vi "checkvisionok.vi"(10 "ResultOut":string[][](array[string])) -> (2 "VisionOK":bool)   [LabVIEW 2019]
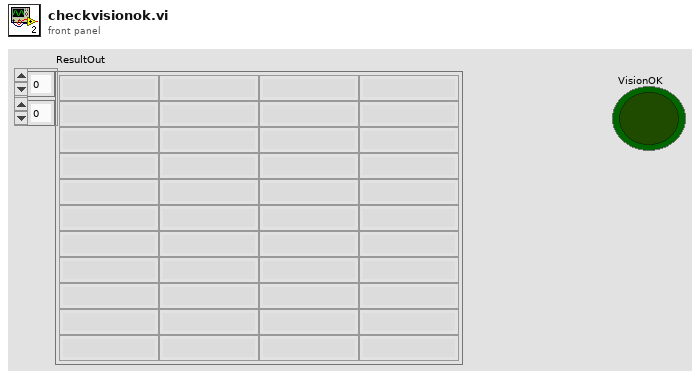
[diagram p1: front panel]
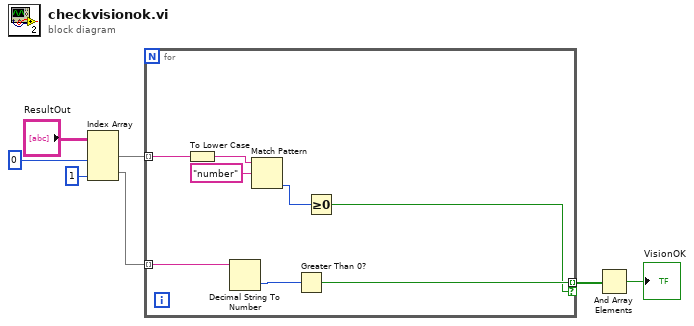
[diagram p0: block diagram]
diagram:
  n1 = Index Array(array="ResultOut", index (col) #1=0 ("disabled index (col)"), index (col) #2=1 ("index (col)")) -> (element #1=w5:string[], element #2=w3:string[])  [unwired: 2 in]
  n2 = for {
    tunnel: w5 -> [w15] mode=indexing
    tunnel: w3 -> [w11] mode=indexing
    tunnel: [w9] -> w2 mode=indexing if=w8
    n3 = To Lower Case(string=w15) -> (all lower case string=w14:string)
    n4 = Decimal String To Number(string=w11) -> (number=w10:i32)  [unwired: 2 in, 1 out]
    n5 = Match Pattern(string=w14, regular expression="number") -> (offset past match=w12:i32)  [unwired: 1 in, 3 out]
    n6 = Greater Than 0?(x=w10) -> (x > 0?=w9:bool)
    n7 = Greater Or Equal To 0?(x=w12) -> (x >= 0?=w8:bool)
  }
  n8 = And Array Elements(Boolean array=w2) -> (logical AND=→"VisionOK":bool)
